vi "lab1.vi"() -> ()   [LabVIEW 2019]
panel:
  in  "stop":bool
  out "Calculations":bool
  out "XY Graph":cluster{dbl[], dbl[]}(graph)
  out "S3":dbl format="%#_20g"
  out "S2":dbl format="%#_20g"
  out "S1":dbl format="%#_18g"
  in  "C":sgl
  in  "B":sgl
  in  "A":sgl
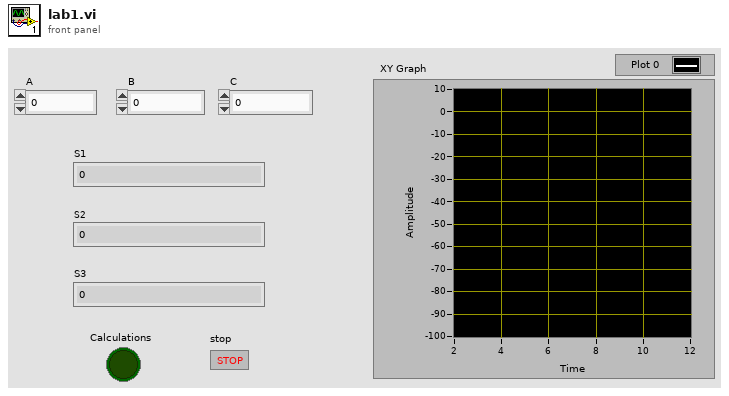
[diagram p1: front panel]
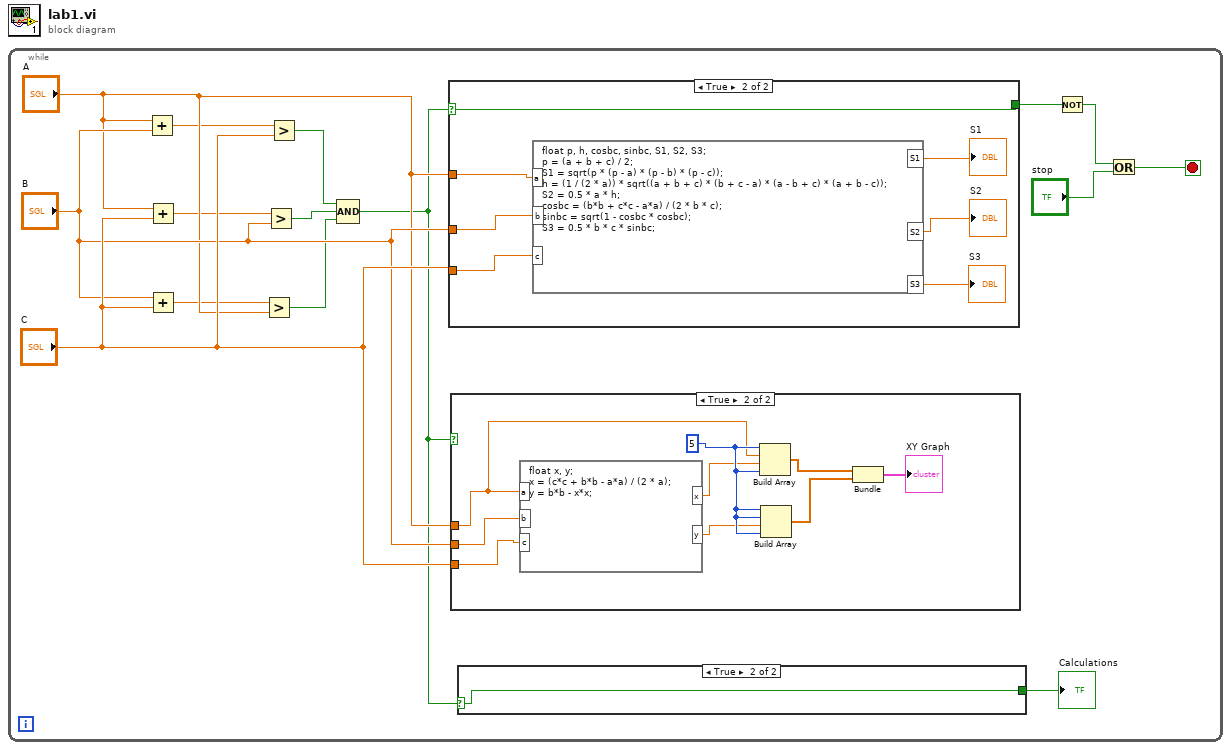
[diagram p0: block diagram]
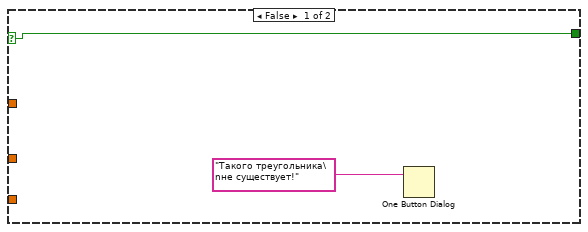
[diagram p4: hidden frame]
diagram:
  n1 = while {
    stop <- w1 stop-if-true
    n2 = Add(x="A", y="B") -> (x+y=w8:sgl)
    n3 = Add(x="A", y="C") -> (x+y=w7:sgl)
    n4 = Add(x="B", y="C") -> (x+y=w9:sgl)
    n5 = Greater?(x=w9, y="A") -> (0:w12:bool)
    n6 = Greater?(x=w7, y="B") -> (0:w11:bool)
    n7 = Greater?(x=w8, y="C") -> (0:w10:bool)
    n8 = Compound Arithmetic op=AND(w10, w11, w12) -> (w6:bool)
    n9 = case shown="True" w6 {
      selector: w6 -> [w27 w35]
      tunnel: [w27 w35] -> w4
      tunnel: "A" -> [_ w34]
      tunnel: "B" -> [_ w33]
      tunnel: "C" -> [_ w32]
      frame False {
        n10 = One Button Dialog(message="Такого треугольника\nне существует!") -> ()  [unwired: 1 in, 1 out]
      }
      frame True {
        n11 = formula code="float p, h, cosbc, sinbc, S1, S2, S3;\np = (a + b + c) / 2;\nS1 = sqrt(p * (p - a) * (p - b) * (p - c));\nh = (1 / (2 * a)) * sqrt((a + b + c) * (b + c - a) * (a - b + c) * (a + b - c));\nS2 = 0.5 * a * h;\ncosbc = (b*b + c*c - a*a) / (2 * b * c);\nsinbc = sqrt(1 - cosbc * cosbc);\nS3 = 0.5 * b * c * sinbc;"("a"=w34, "b"=w33, "c"=w32) -> ("S1"=→"S1":dbl, "S2"=→"S2":dbl, "S3"=→"S3":dbl)
      }
    }
    n12 = case shown="True" w6 {
      tunnel: "A" -> [_ w21]
      tunnel: "B" -> [_ w23]
      tunnel: "C" -> [_ w22]
      frame False {
      }
      frame True {
        w26 = 5
        n13 = formula code="float x, y;\nx = (c*c + b*b - a*a) / (2 * a);\ny = b*b - x*x;"("a"=w21, "b"=w23, "c"=w22) -> ("x"=w24:dbl, "y"=w25:dbl)
        n14 = Build Array(w26, w21, w24, w26) -> (w20:dbl[])
        n15 = Build Array(w26, w26, w25, w26) -> (w19:dbl[])
        n16 = Bundle(w20, w19) -> (→"XY Graph":cluster{dbl[], dbl[]})  [unwired: 1 in]
      }
    }
    n17 = case shown="True" w6 {
      selector: w6 -> [w16 w17]
      tunnel: [w16 w17] -> w5
      frame False {
      }
      frame True {
      }
    }
    "Calculations" <- w5
    n18 = Not(x=w4) -> (.not. x?=w3:bool)
    n19 = Or(x=w3, y="stop") -> (x .or. y?=w1:bool)
  }
